vi "lijnvolgen (SubVI).vi"(8 "snelheid motor rechts":dbl, 9 "snelheid motor links":dbl, 10 "OK Button":bool, 11 "array":dbl[](array[numeric])) -> (0 "output: snelheid motor rechts":dbl, 1 "output: snelheid motor links":dbl, 2 "Boolean":bool)   [LabVIEW 2019]
uses:
  <vilib>/myRIO/Instrument Drivers/Onboard IO/PWM/typedefs/PWM Configuration.ctl
  <vilib>/myRIO/Instrument Drivers/Onboard IO/PWM/PWM.lvlib
  <vilib>/myRIO/Common/Instrument Driver Framework/myRIO v1.0/PWM/typedefs/PWM Channels Enum.ctl
  <vilib>/myRIO/Common/Instrument Driver Framework/Utilities/typedefs/Generic FPGA Reference.ctl
  <vilib>/myRIO/Common/Instrument Driver Framework/Utilities/typedefs/myRIO v1.0 Reference.ctl
  <vilib>/myRIO/Common/Instrument Driver Framework/Utilities/typedefs/Hardware Version Enum.ctl
  <vilib>/myRIO/Common/Instrument Driver Framework/Utilities/typedefs/myRIO Generic Hardware Reference.ctl
  <vilib>/myRIO/Instrument Drivers/Onboard IO/PWM/typedefs/PWM Reference.ctl
  <vilib>/myRIO/Instrument Drivers/Onboard IO/PWM/vis/Set Duty Cycle and Frequency.vi
  <vilib>/userDefined/High Color/nirio_resource_hc.ctl
  <vilib>/myRIO/Common/Instrument Driver Framework/myRIO v1.0/PWM/vis/myRIO v1.1 Open PWM.vi
  <vilib>/myRIO/Instrument Drivers/Onboard IO/PWM/vis/myRIO PWM Open.xnode
  <vilib>/myRIO/Common/Instrument Driver Framework/Utilities/vis/Is FPGA Ref Available.vi
  <vilib>/myRIO/Express VI/Onboard IO/PWM/PWM Express VI.xnode
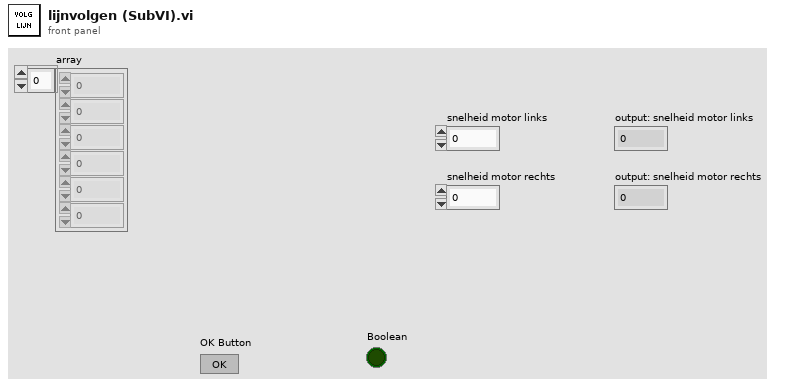
[diagram p1: front panel]
types:
  T1 = typedef "PWM.lvlib/PWM Reference.ctl" = cluster{"myRIO Reference":T2, "PWM Channels Enum":T6, "PWM Configuration":T7}
  T2 = typedef "myRIO Generic Hardware Reference.ctl" = cluster{"myRIO Model":T3, "myRIO Hardware Reference":T4}
  T3 = typedef "Hardware Version Enum.ctl" = enum16{"Unknown", "myRIO-1900", "myRIO-1950", "roboRIO", "NI ELVIS RIO CM", "ELVIS III"}
  T4 = typedef "myRIO v1.0 Reference.ctl" = cluster{"Generic FPGA Reference":T5, "Allow multiple opens":bool}
  T5 = typedef "Generic FPGA Reference.ctl" = refnum<k20>
  T6 = typedef "PWM Channels Enum.ctl" = enum16{"Not Connected", "C/PWM0", "C/PWM1", "A/PWM0", "A/PWM1", "A/PWM2", "A/PWM3", "A/PWM4", "A/PWM5", "A/PWM6", "A/PWM7", "A/PWM8", "A/PWM9", "A/PWM10", "A/PWM11", "A/PWM12", "A/PWM13", "A/PWM14", "A/PWM15", "A/PWM16", "A/PWM17", "A/PWM18", "A/PWM19", "B/PWM0", "B/PWM1", "B/PWM2", "B/PWM3", "B/PWM4", "B/PWM5", "B/PWM6", "B/PWM7", "B/PWM8", "B/PWM9", "B/PWM10", "B/PWM11", "B/PWM12", "B/PWM13", "B/PWM14", "B/PWM15", "B/PWM16", "B/PWM17", "B/PWM18", "B/PWM19", "PWM/PWM0", "PWM/PWM1", "PWM/PWM2", "PWM/PWM3", "PWM/PWM4", "PWM/PWM5", "PWM/PWM6", "PWM/PWM7", "PWM/PWM8", "PWM/PWM9"}
  T7 = typedef "PWM.lvlib/PWM Configuration.ctl" = cluster{"Frequency":dbl, "Duty Cycle":dbl}
  T8 = typedef "nirio_resource_hc.ctl" = tag
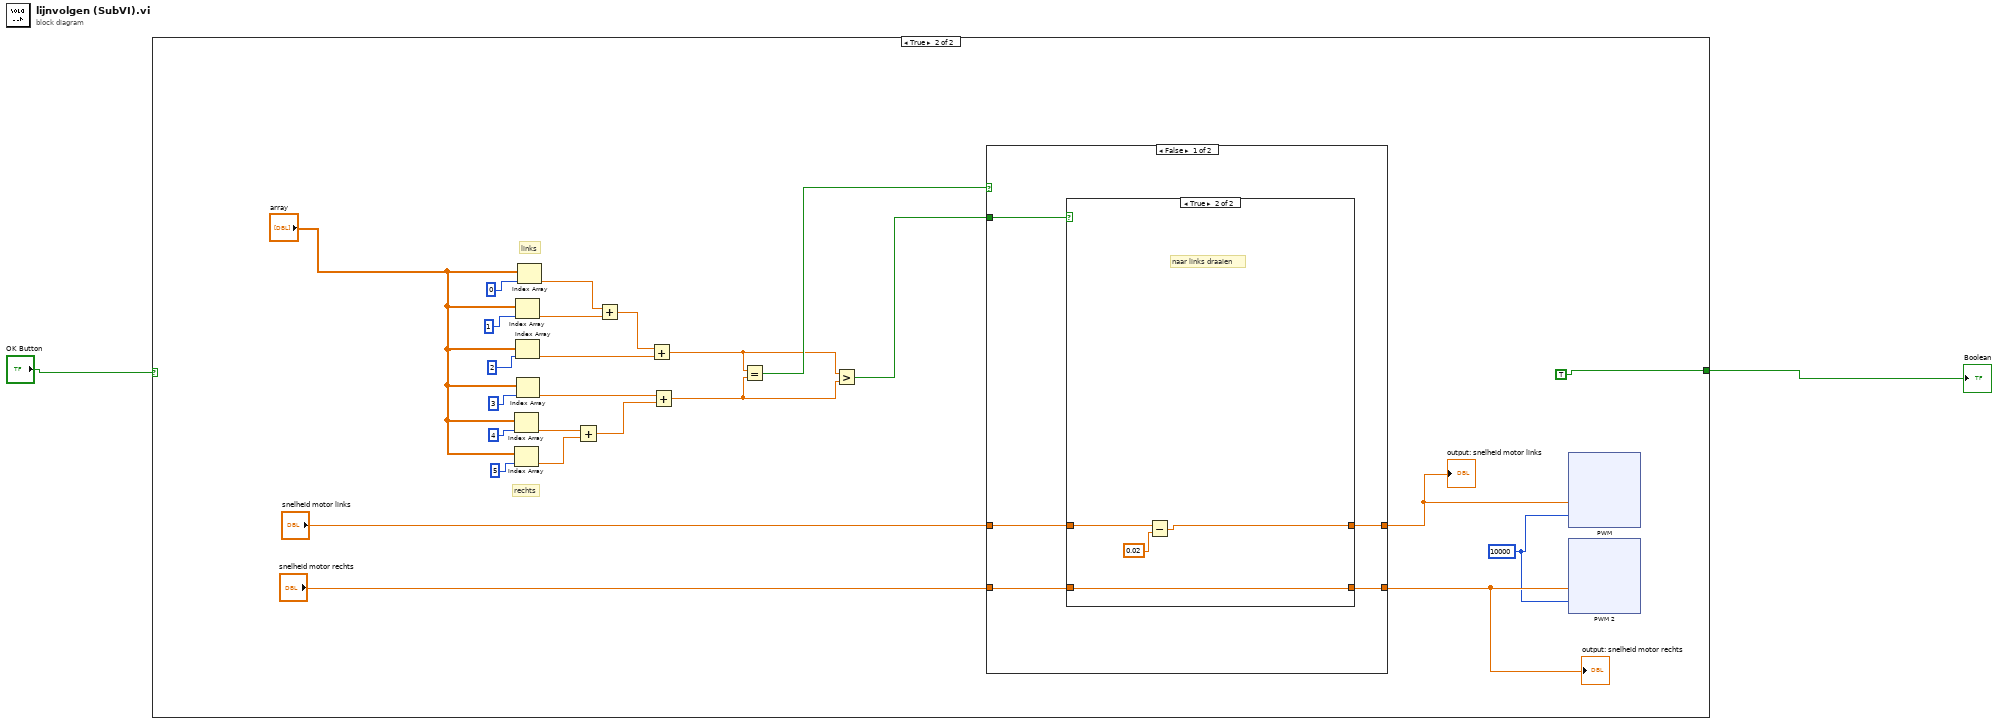
[diagram p0: block diagram]
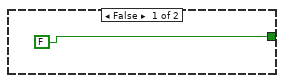
[diagram p2: hidden frame]
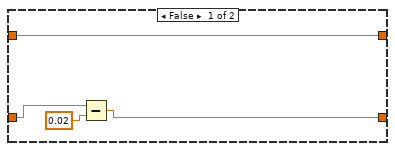
[diagram p3: hidden frame]
diagram:
  n1 = case shown="True" "OK Button" {
    tunnel: [FALSE TRUE] -> w1
    frame False {
    }
    frame True {
      w4 = 10000
      # "rechts"
      # "links"
      n2 = Index Array(array="array", index=4) -> (element=w21:dbl)
      n3 = Index Array(array="array", index=5) -> (element=w22:dbl)
      n4 = Index Array(array="array", index=1) -> (element=w17:dbl)
      n5 = Index Array(array="array", index=2) -> (element=w15:dbl)
      n6 = Index Array(array="array", index=3) -> (element=w20:dbl)
      n7 = Index Array(array="array", index=0) -> (element=w18:dbl)
      n8 = Add(x=w21, y=w22) -> (x+y=w19:dbl)
      n9 = Add(x=w18, y=w17) -> (x+y=w16:dbl)
      n10 = Add(x=w16, y=w15) -> (x+y=w11:dbl)
      n11 = Add(x=w20, y=w19) -> (x+y=w10:dbl)
      n12 = Equal?(x=w11, y=w10) -> (x = y?=w14:bool)
      n13 = Greater?(x=w11, y=w10) -> (0:w9:bool)
      n14 = case shown="False" w14 {
        tunnel: "snelheid motor links" -> [w102 w112]
        tunnel: "snelheid motor rechts" -> [w101 w113]
        tunnel: [w99 w113] -> w6
        tunnel: [w100 w112] -> w5
        tunnel: w9 -> [w103 _]
        frame False {
          n15 = case shown="True" w103 {
            tunnel: w102 -> [w104 w111]
            tunnel: w101 -> [w107 w108]
            tunnel: [w104 w109] -> w100
            tunnel: [w105 w108] -> w99
            frame False {
              n16 = Subtract(x=w107, y=0.02) -> (x-y=w105:dbl)
            }
            frame True {
              # "naar links draaien"
              n17 = Subtract(x=w111, y=0.02) -> (x-y=w109:dbl)
            }
          }
        }
        frame True {
        }
      }
      "output: snelheid motor links" <- w5
      "output: snelheid motor rechts" <- w6
      n18 = xnode "PWM"("Duty Cycle"=w5, "Frequency [Hz]"=w4) -> ()  [unwired: 1 in, 1 out]
      n19 = xnode "PWM 2"("Duty Cycle"=w6, "Frequency [Hz]"=w4) -> ()  [unwired: 1 in, 1 out]
    }
  }
  "Boolean" <- w1
